vi "templogger.vi"() -> ()   [LabVIEW 2017]
panel:
  out "error out":errorcluster
  in  "file (use dialog)":path
  out "Temperature":dbl
  out "Time":timestamp
  in  "Data request every nth second":dbl
  in  "stop":bool
  out "Date & Temp String":string
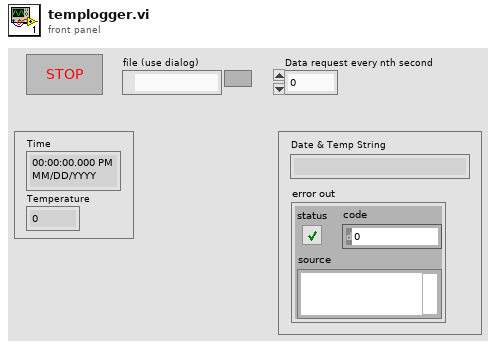
[diagram p1: front panel]
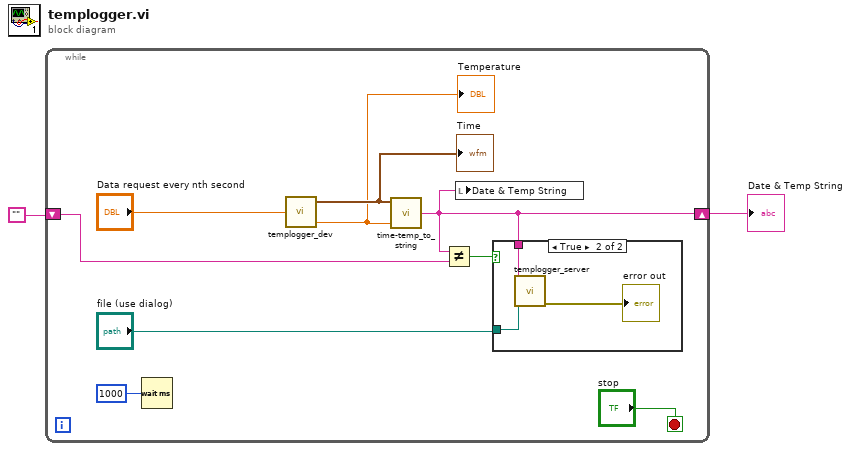
[diagram p0: block diagram]
diagram:
  n1 = while {
    shift-right: [w7] -> w2
    shift-left: "" -> [w8]
    stop <- "stop" stop-if-true
    n2 = Wait (ms)(milliseconds to wait=u32 1000) -> ()  [unwired: 1 out]
    n3 = call "templogger_dev.vi"("Seconds"="Data request every nth second") -> ("Temperature"=w3:dbl, "Time"=w4:timestamp)  [unwired: 3 in]
    "Time" <- w4
    "Temperature" <- w3
    n4 = call "time-temp_to_string.vi"("Time"=w4, "Temperature"=w3) -> ("String"=w7:string)  [unwired: 5 in]
    n5 = Not Equal?(x=w7, y=w8) -> (x != y?=w9:bool)
    n6 = local write "Date & Temp String"(w7) -> ()
    n7 = case shown="True" w9 {
      tunnel: "file (use dialog)" -> [_ w13]
      tunnel: w7 -> [_ w12]
      frame False {
      }
      frame True {
        n8 = call "templogger_server.vi"("Input String"=w12, "file (use dialog)"=w13) -> ("error out"=→"error out":errorcluster)  [unwired: 9 in]
      }
    }
  }
  "Date & Temp String" <- w2
